vi "Open Audio File Write.vi"   [LabVIEW 2020, in "G-Audio.lvlib"]
uses:
  G-Audio.lvlib
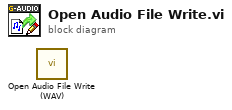
[diagram p0: block diagram]
diagram:
  n1 = call "Open Audio File Write (WAV).vi"() -> ()  [unwired: 10 in, 2 out]
